vi "Inventory Path Global.vi"() -> ()   [LabVIEW 2013]
panel:
  in  "Inventory Path":path=path "C:/Users/alecjcook/Documents/GitHub/LabVIEW/Electronics/Inventory/HomeLabInv.txt"
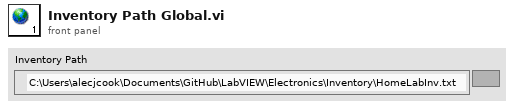
[diagram p1: front panel]
diagram:
